vi "Recursive Test.vi"() -> ()   [LabVIEW 2018]
panel:
  in  "#Elements":i32=3
  in  "Input":string="1933\n1963\n1924\n1832\n1949\n1826\n1681\n1548\n1881\n1973\n1558\n1979\n1803\n1975\n1867\n1934\n1986\n1220\n1878\n1985\n2006\n1535\n1522\n1884\n1380\n1922\n1905\n1582\n1456\n1877\n1959\n1953\n634\n1875\n366\n1968\n1887\n1848\n1779\n1894\n1606\n1429\n1900\n1309\n2007\n1944\n1901\n1559\n1484\n1996\n1837\n1892\n1989\n1684\n1952\n1990\n1974\n1890\n1883\n1993\n1592\n1889\n1735\n1577\n1568\n1957\n1980\n1537\n1992\n1950\n1836\n1397\n1660\n2010\n1627\n1991\n1888\n107\n1977\n1898\n1532\n1726\n1899\n1960\n1962\n2000\n1903\n1937\n1931\n1895\n1868\n1600\n1926\n1946\n1964\n1956\n1915\n1506\n1580\n1984\n1870\n2008\n1885\n1503\n1927\n841\n1997\n2002\n1869\n1874\n1906\n1911\n508\n1718\n1961\n1909\n1914\n1940\n1879\n1965\n1929\n1932\n1579\n1902\n1783\n1983\n166\n1972\n2003\n2005\n1918\n1893\n1427\n1945\n1982\n1847\n1425\n1941\n1958\n1842\n1928\n1840\n1789\n1654\n1665\n1387\n1908\n1891\n1873\n1839\n1943\n1616\n1490\n144\n1981\n1988\n1853\n1994\n42\n1954\n1762\n1792\n1896\n1907\n1976\n1886\n1971\n1998\n1912\n1967\n1857\n1951\n1925\n1921\n1518\n1593\n2004\n1999\n1571\n1923\n463\n1897\n1861\n1467\n1920\n1504\n2009\n1942\n1995\n1947\n1872\n1969\n1910\n1955\n1939\n1966\n1687\n1827\n675\n1520"
  out "Numeric":dbl format="%#.0f"
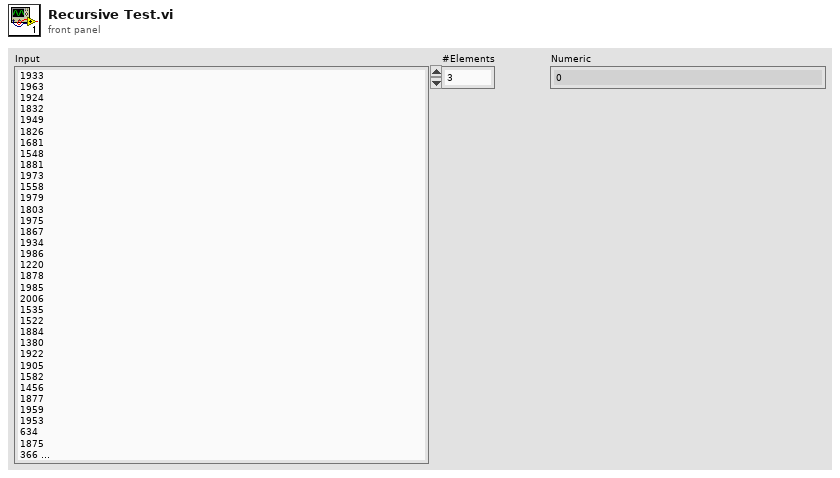
[diagram p1: front panel]
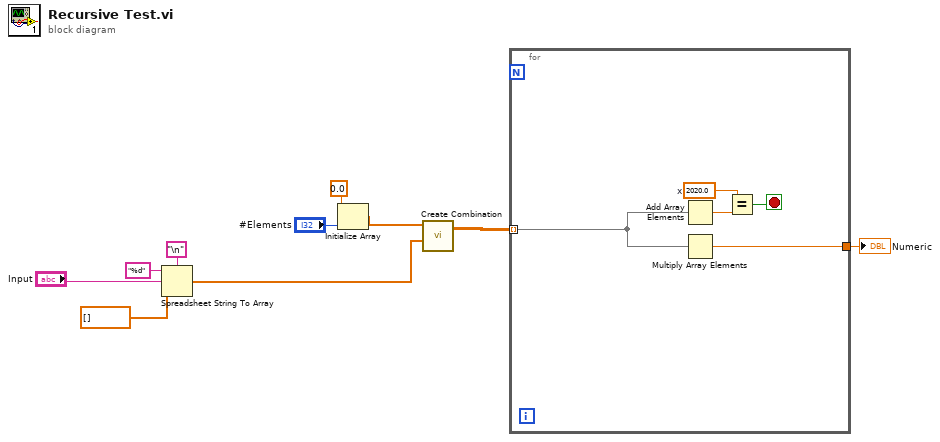
[diagram p0: block diagram]
diagram:
  n1 = Spreadsheet String To Array(delimiter (Tab)="\n", format string="%d", spreadsheet string="Input", array type (2D Dbl)=dbl[] []) -> (array=w3:dbl[])
  n2 = Initialize Array(0.0, "#Elements") -> (w8:dbl[])
  n3 = call "Create Combination.vi"("Array"=w3, "Temp Combination"=w8) -> ("Combinations Out"=w7:dbl[][])  [unwired: 9 in]
  n4 = for {
    tunnel: w7 -> [w15] mode=indexing
    tunnel: [w11] -> w2
    stop <- w12 stop-if-true
    w13 = 2020.0  # x
    n5 = Add Array Elements(numeric array=w15) -> (sum=w14:dbl)
    n6 = Multiply Array Elements(1:w15) -> (0:w11:dbl)
    n7 = Equal?(x=w13, y=w14) -> (x = y?=w12:bool)
  }
  "Numeric" <- w2
